vi "Teleop_sav.vi"(10 "Match Info":T1={"Autonomous Elapsed Seconds"=0.0, "TeleOp Elapsed Seconds"=0.0, "Disabled Elapsed Seconds"=0.0, "Visited Autonomous"=FALSE, "Visited TeleOp"=FALSE, "Visited Disabled"=FALSE, "Autonomous Settings"={"Autonomous Style"=enum."Independent", "VI Refnum"=refnum}}, 11 "Call Context":T2) -> ()   [LabVIEW 2014]
doc: "This VI is called for each TeleOp packet received from the DS where the robot is not disabled. It is often used to read from the joysticks and update I/O or to update setpoints for timed control loops. It should complete and return within 20 milliseconds or it may miss DS packets."
uses:
  <vilib>/Rock Robotics/WPI/DriverStation/WPI_DriverStationDerivedRobotMode.ctl
  <vilib>/Rock Robotics/WPI/DriverStation/WPI_DriverStationMatch Info.ctl
  <vilib>/Rock Robotics/WPI/RobotDrive/WPI_RobotDriveGetSetRefNum.vi
  <vilib>/Rock Robotics/WPI/Joystick/WPI_JoystickGetSetRefNum.vi
  <vilib>/Rock Robotics/Network Tables/SD Write Boolean Array.vi
  <vilib>/Rock Robotics/Network Tables/SD Write Boolean.vi
  <vilib>/Rock Robotics/Network Tables/SD Read Number.vi
  <vilib>/Rock Robotics/Network Tables/SD Write Number.vi
  <vilib>/Rock Robotics/WPI/Compressor/WPI_CompressorGetSetRefNum.vi
  <vilib>/Rock Robotics/WPI/Solenoid/Deprecated/WPI_SolenoidSetBool.vi
  <vilib>/Rock Robotics/Network Tables/SD Read Boolean.vi
  <vilib>/addons/control/pid/pid.llb/PID (DBL).vi
  <vilib>/Rock Robotics/WPI/RobotDrive/WPI_RobotDriveMecanumDrive_Cartesian.vi
  <vilib>/Rock Robotics/Network Tables/SD Write Numeric Array.vi
  <vilib>/addons/control/pid/NI_PID_pid.lvlib
panel:
  in  "Lift Encoder Target":dbl
  out "all currents (A)":dbl[](array[numeric])
  out "input current (A)":dbl
  out "input voltage (V)":dbl
  out "In-Range":bool
  out "Lift Stopped":bool
  out "Lift Direction":bool
  out "Lift Encoder Distance":dbl
  out "Lift Encoder Rate":dbl
  out "Bottom Limit":bool
  out "Top Limit":bool
  out "Wheel Stopped":bool
  out "Wheel Direction":bool
  out "Wheel Encoder Distance":dbl
  out "Wheel Encoder Rate":dbl
  out "Lift Motor Speed":dbl
  out "Angle":dbl(knob) scale=0.0..360.0
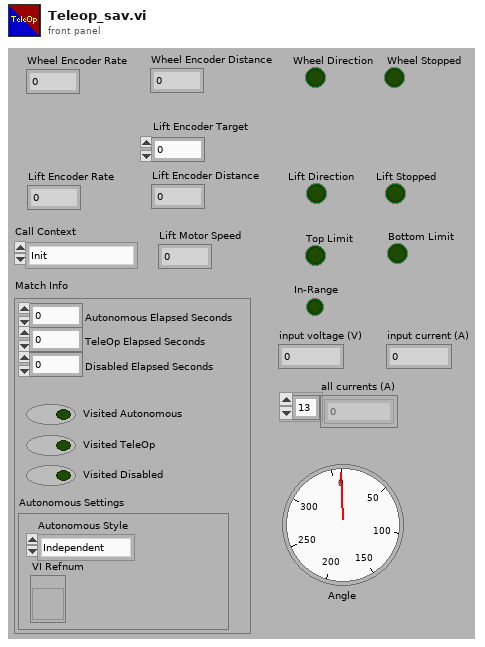
[diagram p1: front panel]
types:
  T1 = typedef "WPI_DriverStationMatch Info.ctl" = cluster{"Autonomous Elapsed Seconds":dbl, "TeleOp Elapsed Seconds":dbl, "Disabled Elapsed Seconds":dbl, "Visited Autonomous":bool, "Visited TeleOp":bool, "Visited Disabled":bool, "Autonomous Settings":cluster{"Autonomous Style":enum16{"Iterative", "Independent"}, "VI Refnum":refnum<vi>}}
  T2 = typedef "WPI_DriverStationDerivedRobotMode.ctl" = enum16{"Init", "Execute", "Stop"}
  T3 = cluster{"proportional gain (Kc)":dbl, "integral time (Ti, min)":dbl, "derivative time (Td, min)":dbl}
  T4 = typedef "WPI_JoystickDevRef.ctl" = cluster{"Device":T5}
  T5 = typedef "WPI_JoystickDeviceEnum.ctl" = enum16{"USB 0", "USB 1", "USB 2", "USB 3", "USB 4", "USB 5"}
  T6 = typedef "WPI_GyroDevRef.ctl" = cluster{"DevStatus":errorcluster, "Analog Module":T7, "Analog Channel":T8, "Offset":dbl, "Gain (VoltsPerDegree/Second)":dbl}
  T7 = typedef "FPGA_TypedefAnalogModule.ctl" = enum16{"Controller 1"}
  T8 = typedef "FPGA_AIChannel.ctl" = enum8{"AI 0", "AI 1", "AI 2", "AI 3", "AI MXP 0", "AI MXP 1", "AI MXP 2", "AI MXP 3", "Invalid"}
  T9 = typedef "WPI_EncoderDevRef.ctl" = cluster{"DevStatus":errorcluster, "EncoderIndex":T10, "CounterIndex":T11, "DistancePerCount":dbl, "Decoding Type":T12}
  T10 = typedef "FPGA_EncoderIdx.ctl" = enum8{"Enc 0", "Enc 1", "Enc 2", "Enc 3", "Enc 4", "Enc 5", "Enc 6", "Enc 7", "Invalid"}
  T11 = typedef "FPGA_CounterCtrSystemIndex.ctl" = enum8{"Ctr 0", "Ctr 1", "Ctr 2", "Ctr 3", "Ctr 4", "Ctr 5", "Ctr 6", "Ctr 7", "Invalid"}
  T12 = typedef "WPI_EncoderType.ctl" = enum16{"1x", "2x", "4x"}
  T13 = typedef "WPI_SolenoidDevRef.ctl" = cluster{"DevStatus":errorcluster, "Pneumatics Control Module":u8, "Forward Solenoid Channel":T14, "Reverse Solenoid Channel":T14}
  T14 = typedef "WPI_SolenoidChannel.ctl" = enum8{"Solenoid 0", "Solenoid 1", "Solenoid 2", "Solenoid 3", "Solenoid 4", "Solenoid 5", "Solenoid 6", "Solenoid 7", "Invalid"}
  T15 = cluster{"Buttons[0]":bool, "Buttons[1]":bool, "Buttons[2]":bool, "Buttons[3]":bool, "Buttons[4]":bool, "Buttons[5]":bool, "Buttons[6]":bool, "Buttons[7]":bool, "Buttons[8]":bool}
  T16 = typedef "WPI_RobotDriveDevRef.ctl" = cluster{"DevStatus":errorcluster, "Motors[]":T17[], "Square Inputs":bool, "Max Output":dbl}
  T17 = typedef "WPI_MotorControlDeviceRef.ctl" = cluster{"DeviceStatus":errorcluster, "Type":T18, "PWM":cluster{"Controller":T19, "PWM Channel":T20, "DeadBand":T21}, "CAN":cluster{"Device Number":u8, "Control Mode":T22, "Semaphore":T23, "Max Vout":dbl, "TalonSRX Control Mode":T24}, "Invert":bool, "TransformRef":T25, "InvTransformRef":T25}
  T18 = typedef "WPI_MotorControlType.ctl" = enum16{"PWM", "CAN", "CANTalonSRX"}
  T19 = typedef "FPGA_TypedefDigitalModule.ctl" = enum16{"Controller 1"}
  T20 = typedef "FPGA_DIOPWMChannel.ctl" = enum8{"PWM 0", "PWM 1", "PWM 2", "PWM 3", "PWM 4", "PWM 5", "PWM 6", "PWM 7", "PWM 8", "PWM 9", "PWM MXP 0", "PWM MXP 1", "PWM MXP 2", "PWM MXP 3", "PWM MXP 4", "PWM MXP 5", "PWM MXP 6", "PWM MXP 7", "PWM MXP 8", "PWM MXP 9", "Invalid"}
  T21 = typedef "WPI_PWMDeadband.ctl" = cluster{"Name":string, "maxPositivePwm":i32, "minPositivePwm":i32, "centerPwm":i32, "maxNegativePwm":i32, "minNegativePwm":i32, "angularRange":u16}
  T22 = typedef "WPI_CANJaguar_ControlMode.ctl" = enum8{"Percent VBus", "Current", "Speed", "Position", "Voltage"}
  T23 = typedef "Semaphore RefNum" = refnum<k1>
  T24 = typedef "WPI_CANTalonSRX_APIControlMode.ctl" = enum8{"Percent VBus", "Speed", "Position", "Slave", "Unchanged / Invalid"}
  T25 = typedef "WPI_PWMTransform_ConPane.ctl" = refnum<vi>
  T26 = typedef "WPI_SwitchDevRef.ctl" = cluster{"DevStatus":errorcluster, "DIO Channel":T27, "Controller":T19, "CntIndex":T11, "Normally Closed":bool}
  T27 = typedef "FPGA_DIOChannel.ctl" = enum8{"DIO 0", "DIO 1", "DIO 2", "DIO 3", "DIO 4", "DIO 5", "DIO 6", "DIO 7", "DIO 8", "DIO 9", "DIO MXP 0", "DIO MXP 1", "DIO MXP 2", "DIO MXP 3", "DIO MXP 4", "DIO MXP 5", "DIO MXP 6", "DIO MXP 7", "DIO MXP 8", "DIO MXP 9", "DIO MXP 10", "DIO MXP 11", "DIO MXP 12", "DIO MXP 13", "DIO MXP 14", "DIO MXP 15", "Invalid"}
  T28 = cluster{"X":dbl, "Y":dbl, "Angle":dbl, "Magnitude":dbl}
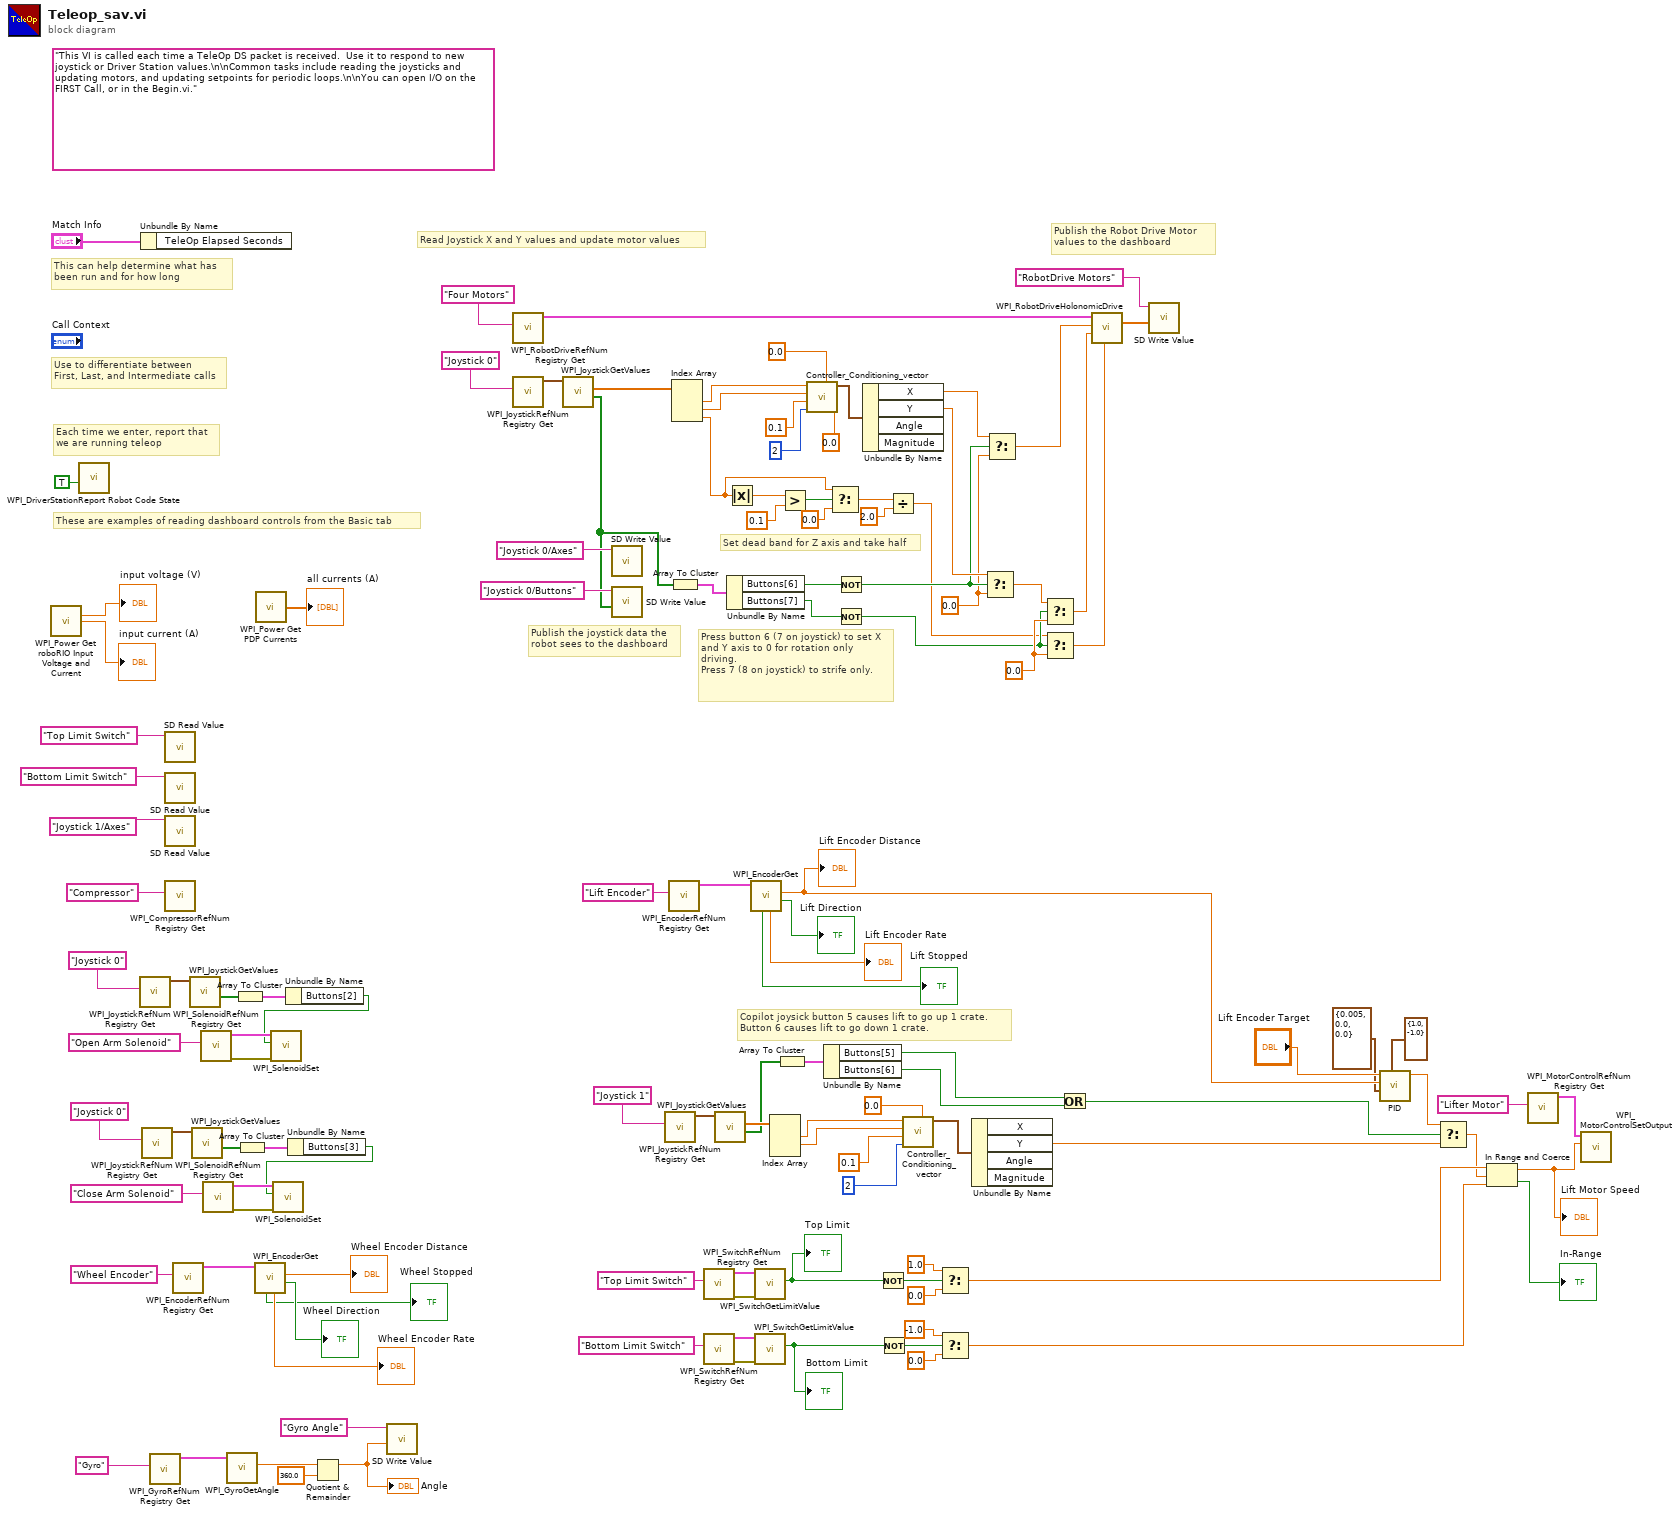
[diagram p0: block diagram]
diagram:
  w30 = 0.0 ("f")
  w82 = 0.0
  (unwired) "This VI is called each time a TeleOp DS packet is received.  Use it to respond to new joystick or Driver Station values.\n\nCommon tasks include reading the joysticks and updating motors, and updating setpoints for periodic loops.\n\nYou can open I/O on the FIRST Call, or in the Begin.vi."
  # "Copilot joysick button 5 causes lift to go up 1 crate.\nButton 6 causes lift to go down 1 crate."
  # "Set dead band for Z axis and take half"
  # "Press button 6 (7 on joystick) to set X and Y axis to 0 for rotation only driving.\nPress 7 (8 on joystick) to strife only."
  # "These are examples of reading dashboard controls from the Basic tab"
  # "Publish the Robot Drive Motor\nvalues to the dashboard"
  # "Publish the joystick data the\nrobot sees to the dashboard"
  # "Each time we enter, report that\nwe are running teleop"
  # "Use to differentiate between\nFirst, Last, and Intermediate calls"
  # "This can help determine what has\nbeen run and for how long"
  # "Read Joystick X and Y values and update motor values"
  n1 = call <vilib>:"WPI_Power Get roboRIO Input Voltage and Current.vi"() -> ("roboRIO input voltage (V)"=→"input voltage (V)":dbl, "roboRIO input current (A)"=→"input current (A)":dbl)  [unwired: 13 in, 1 out]
  n2 = call <vilib>:"WPI_DriverStationReport Robot Code State.vi"("TeleOp"=TRUE ("Autonomous")) -> ()  [unwired: 10 in, 1 out]
  n3 = call <vilib>:"WPI_JoystickRefNum Registry Get.vi"("refnum name"="Joystick 0") -> ("JoystickDevRef"=w71:T4)  [unwired: 1 in, 9 out]
  n4 = Unbundle By Name("Match Info") -> ()  [unwired: 1 out]
  n5 = call <vilib>:"WPI_JoystickRefNum Registry Get.vi"("refnum name"="Joystick 0") -> ("JoystickDevRef"=w58:T4)  [unwired: 1 in, 9 out]
  n6 = call <vilib>:"WPI_GyroRefNum Registry Get.vi"("refnum name"="Gyro") -> ("GyroDevRef"=w103:T6)  [unwired: 9 in, 1 out]
  n7 = call-poly <vilib>:"SD Read Value.vi"("Name"="Top Limit Switch" ("refnum name")) -> ()  [unwired: 8 in, 3 out]
  n8 = call-poly <vilib>:"SD Read Value.vi"("Name"="Bottom Limit Switch" ("refnum name")) -> ()  [unwired: 8 in, 3 out]
  n9 = call-poly <vilib>:"SD Read Value.vi"("Name"="Joystick 1/Axes" ("refnum name")) -> ()  [unwired: 8 in, 3 out]
  n10 = call <vilib>:"WPI_CompressorRefNum Registry Get.vi"("refnum name"="Compressor") -> ()  [unwired: 9 in, 2 out]
  n11 = call <vilib>:"WPI_EncoderRefNum Registry Get.vi"("refnum name"="Wheel Encoder") -> ("EncoderDevRef"=w78:T9)  [unwired: 9 in, 1 out]
  n12 = call <vilib>:"WPI_JoystickGetValues.vi"("JoystickDevRef"=w71) -> ("Buttons"=w67:bool[])  [unwired: 6 in, 4 out]
  n13 = call <vilib>:"WPI_JoystickGetValues.vi"("JoystickDevRef"=w58) -> ("Buttons"=w54:bool[])  [unwired: 6 in, 4 out]
  n14 = call <vilib>:"WPI_SolenoidRefNum Registry Get.vi"("refnum name"="Open Arm Solenoid") -> ("error out"=w70:errorcluster, "SolenoidDevRef"=w69:T13)  [unwired: 9 in]
  n15 = call <vilib>:"WPI_SolenoidRefNum Registry Get.vi"("refnum name"="Close Arm Solenoid") -> ("error out"=w57:errorcluster, "SolenoidDevRef"=w56:T13)  [unwired: 9 in]
  n16 = call <vilib>:"WPI_GyroGetAngle.vi"("GyroDevRef"=w103) -> ("Angle"=w100:dbl)  [unwired: 7 in, 3 out]
  n17 = Array To Cluster(array=w67) -> (cluster=w66:T15)
  n18 = Array To Cluster(array=w54) -> (cluster=w53:T15)
  n19 = call <vilib>:"WPI_EncoderGet.vi"("EncoderDevRef"=w78) -> ("Direction"=→"Wheel Direction":bool, "Distance"=→"Wheel Encoder Distance":dbl, "Rate"=→"Wheel Encoder Rate":dbl, "Stopped"=→"Wheel Stopped":bool)  [unwired: 5 in, 2 out]
  n20 = call <vilib>:"WPI_Power Get PDP Currents.vi"() -> ("all currents (A)"=→"all currents (A)":dbl[])  [unwired: 13 in, 2 out]
  n21 = Unbundle By Name(w66) -> ("Buttons[2]"=w39:bool)
  n22 = call-poly <vilib>:"WPI_SolenoidSet.vi"("error in (no error)"=w70, "Value"=w39, "SolenoidDevRef"=w69) -> ()  [unwired: 7 in, 2 out]
  n23 = Unbundle By Name(w53) -> ("Buttons[3]"=w52:bool)
  n24 = call-poly <vilib>:"WPI_SolenoidSet.vi"("error in (no error)"=w57, "Value"=w52, "SolenoidDevRef"=w56) -> ()  [unwired: 7 in, 2 out]
  n25 = Quotient & Remainder(x=w100, y=360.0) -> (x-y*floor(x/y)=w25:dbl)  [unwired: 1 out]
  "Angle" <- w25
  n26 = call-poly <vilib>:"SD Write Value.vi"("Numeric"=w25, "Name"="Gyro Angle") -> ()  [unwired: 8 in, 2 out]
  n27 = call <vilib>:"WPI_RobotDriveRefNum Registry Get.vi"("refnum name"="Four Motors") -> ("RobotDriveDevRef"=w119:T16)  [unwired: 1 in, 9 out]
  n28 = call <vilib>:"WPI_JoystickRefNum Registry Get.vi"("refnum name"="Joystick 0") -> ("JoystickDevRef"=w117:T4)  [unwired: 1 in, 9 out]
  n29 = call <vilib>:"WPI_JoystickGetValues.vi"("JoystickDevRef"=w117) -> ("Buttons"=w87:bool[], "Axes"=w110:dbl[])  [unwired: 6 in, 3 out]
  n30 = call-poly <vilib>:"SD Write Value.vi"("Name"="Joystick 0/Axes") -> ()  [unwired: 9 in, 2 out]
  n31 = call-poly <vilib>:"SD Write Value.vi"("Boolean Array"=w87, "Name"="Joystick 0/Buttons") -> ()  [unwired: 8 in, 2 out]
  n32 = call <vilib>:"WPI_JoystickRefNum Registry Get.vi"("refnum name"="Joystick 1") -> ("JoystickDevRef"=w97:T4)  [unwired: 1 in, 9 out]
  n33 = call <vilib>:"WPI_EncoderRefNum Registry Get.vi"("refnum name"="Lift Encoder") -> ("EncoderDevRef"=w44:T9)  [unwired: 9 in, 1 out]
  n34 = Array To Cluster(array=w87) -> (cluster=w86:T15)
  n35 = Index Array(array=w110) -> (element #1=w109:dbl, element #2=w108:dbl, element #3=w19:dbl)  [unwired: 3 in]
  n36 = call <vilib>:"WPI_SwitchRefNum Registry Get.vi"("refnum name"="Top Limit Switch") -> ("error out"=w63:errorcluster, "SwitchDevRef"=w64:T26)  [unwired: 9 in]
  n37 = call <vilib>:"WPI_SwitchRefNum Registry Get.vi"("refnum name"="Bottom Limit Switch") -> ("error out"=w60:errorcluster, "SwitchDevRef"=w61:T26)  [unwired: 9 in]
  n38 = call <vilib>:"WPI_JoystickGetValues.vi"("JoystickDevRef"=w97) -> ("Buttons"=w13:bool[], "Axes"=w96:dbl[])  [unwired: 6 in, 3 out]
  n39 = Absolute Value(x=w19) -> (abs(x)=w21:dbl)
  n40 = Unbundle By Name(w86) -> ("Buttons[6]"=w84:bool, "Buttons[7]"=w31:bool)
  n41 = call <vilib>:"WPI_EncoderGet.vi"("EncoderDevRef"=w44) -> ("Direction"=→"Lift Direction":bool, "Distance"=w4:dbl, "Rate"=→"Lift Encoder Rate":dbl, "Stopped"=→"Lift Stopped":bool)  [unwired: 5 in, 2 out]
  "Lift Encoder Distance" <- w4
  n42 = call <vilib>:"WPI_SwitchGetLimitValue.vi"("error in (no error)"=w63, "SwitchDevRef"=w64) -> ("Switch Pressed"=w35:bool)  [unwired: 7 in, 2 out]
  "Top Limit" <- w35
  n43 = call <vilib>:"WPI_SwitchGetLimitValue.vi"("error in (no error)"=w60, "SwitchDevRef"=w61) -> ("Switch Pressed"=w33:bool)  [unwired: 7 in, 2 out]
  "Bottom Limit" <- w33
  n44 = Index Array(array=w96) -> (element #1=w95:dbl, element #2=w94:dbl)  [unwired: 3 in, 1 out]
  n45 = Array To Cluster(array=w13) -> (cluster=w12:T15)
  n46 = Greater?(x=w21, y=0.1) -> (0:w23:bool)
  n47 = call "Controller_Conditioning_vector.vi"("Angular Offset\n(-180 to 180 or 0 to 360)"=0.0 ("Angular Offset\n(-180 to 180 or 0 to 360)"), "Min Output(0 to 1)"=0.0, "Enum"=2, "Dead Zone(0 to 1)"=0.1, "Y(-1 to 1)"=w108, "X(-1 to 1)"=w109) -> ("output cluster"=w107:T28)  [unwired: 5 in]
  n48 = Unbundle By Name(w12) -> ("Buttons[5]"=w7:bool, "Buttons[6]"=w8:bool)
  n49 = Select(t=w19, s=w23, f=0.0) -> (s? t:f=w18:dbl)
  n50 = Not(x=w84) -> (.not. x?=w83:bool)
  n51 = Not(x=w31) -> (.not. x?=w29:bool)
  n52 = Unbundle By Name(w107) -> ("X"=w80:dbl, "Y"=w85:dbl)  [unwired: 2 out]
  n53 = Not(x=w35) -> (.not. x?=w34:bool)
  n54 = Not(x=w33) -> (.not. x?=w32:bool)
  n55 = Divide(x=w18, y=2.0) -> (x/y=w17:dbl)
  n56 = call "Controller_Conditioning_vector.vi"("Min Output(0 to 1)"=0.0, "Enum"=2, "Dead Zone(0 to 1)"=0.1, "Y(-1 to 1)"=w94, "X(-1 to 1)"=w95) -> ("output cluster"=w93:T28)  [unwired: 6 in]
  n57 = Select(t=1.0, s=w34, f=0.0 ("t")) -> (s? t:f=w47:dbl)
  n58 = Select(t=-1.0, s=w32, f=0.0 ("t")) -> (s? t:f=w46:dbl)
  n59 = Unbundle By Name(w93) -> ("Y"=w10:dbl)  [unwired: 3 out]
  n60 = Select(t=w85, s=w83, f=w82) -> (s? t:f=w28:dbl)
  n61 = Select(t=w80, s=w83, f=w82) -> (s? t:f=w81:dbl)
  n62 = Select(t=w28, s=w29, f=w30) -> (s? t:f=w27:dbl)
  n63 = Select(t=w17, s=w29, f=w30) -> (s? t:f=w26:dbl)
  n64 = Or(x=w7, y=w8) -> (x .or. y?=w9:bool)
  n65 = call-poly <vilib>:"WPI_RobotDriveHolonomicDrive.vi"("Rotation"=w26, "Y"=w27, "X"=w81, "RobotDriveDevRef"=w119) -> ("Motor Values"=w111:dbl[])  [unwired: 5 in, 2 out]
  n66 = call-poly <vilib>:"SD Write Value.vi"("Numeric Array"=w111, "Name"="RobotDrive Motors") -> ()  [unwired: 8 in, 2 out]
  n67 = call-poly <vilib>:"PID.vi"("output range"=cluster{"output high":dbl, "output low":dbl} {"output high"=1.0, "output low"=-1.0}, "PID gains"=T3 {"proportional gain (Kc)"=0.005, "integral time (Ti, min)"=0.0, "derivative time (Td, min)"=0.0}, "process variable"=w4, "setpoint"="Lift Encoder Target") -> ("output"=w6:dbl)  [unwired: 6 in, 1 out]
  n68 = Select(t=w6, s=w9, f=w10) -> (s? t:f=w11:dbl)
  n69 = In Range and Coerce(upper limit=w47, x=w11, lower limit=w46) -> (coerced(x)=w36:dbl, In Range?=→"In-Range":bool)
  "Lift Motor Speed" <- w36
  n70 = call <vilib>:"WPI_MotorControlRefNum Registry Get.vi"("refnum name"="Lifter Motor") -> ("MotorControlDevRef"=w89:T17)  [unwired: 9 in, 1 out]
  n71 = call <vilib>:"WPI_MotorControlSetOutput.vi"("Output"=w36, "MotorControlDevRef"=w89) -> ()  [unwired: 7 in, 3 out]
